vi "GlobalStop.vi"() -> ()   [LabVIEW 2013]
panel:
  in  "Stopp":bool
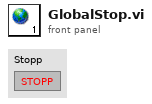
[diagram p1: front panel]
diagram:
